vi "PulseIntervalHistogram_Relative.vi"(7 "Binary array reference":bool[](array[boolean]), 8 "Pulse count in":u64, 9 "No of SI bins":dbl=50.0, 11 "Binary array probe":bool[](array[boolean])) -> (0 "Pulse count out":u64, 1 "Pulse histogram":T1(graph), 2 "Pulse length histogram":T1(graph), 3 "Pulse period histogram":T1(graph))   [LabVIEW 2012]
uses:
  <vilib>/Analysis/NI_AALPro.lvlib
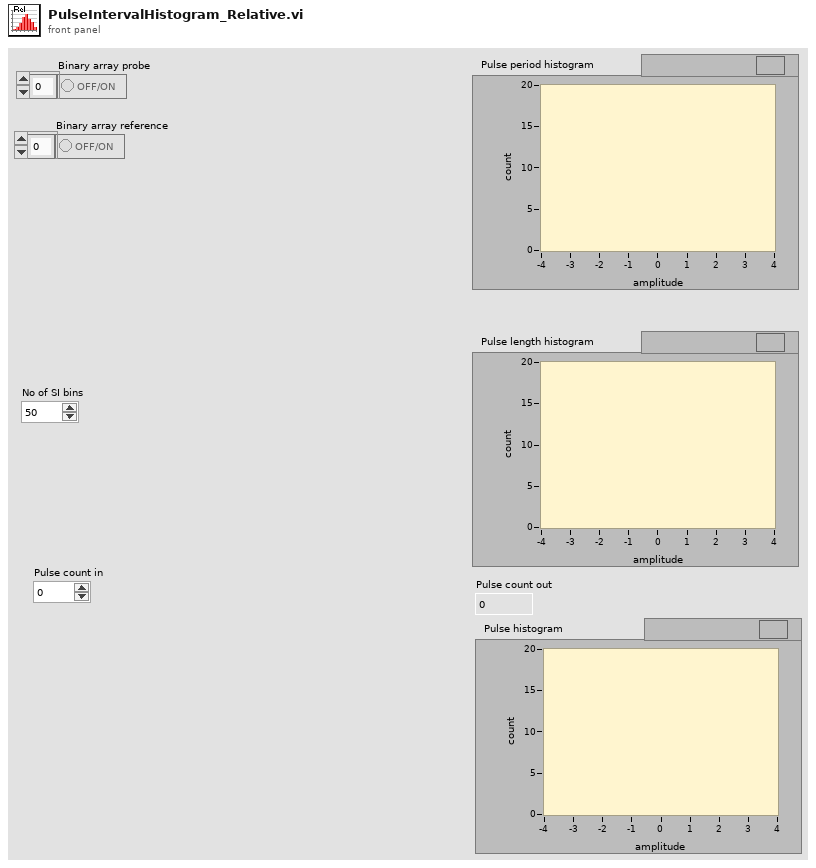
[diagram p1: front panel]
types:
  T1 = cluster{"X Values":dbl[], "Histogram: h(x)":i32[]}
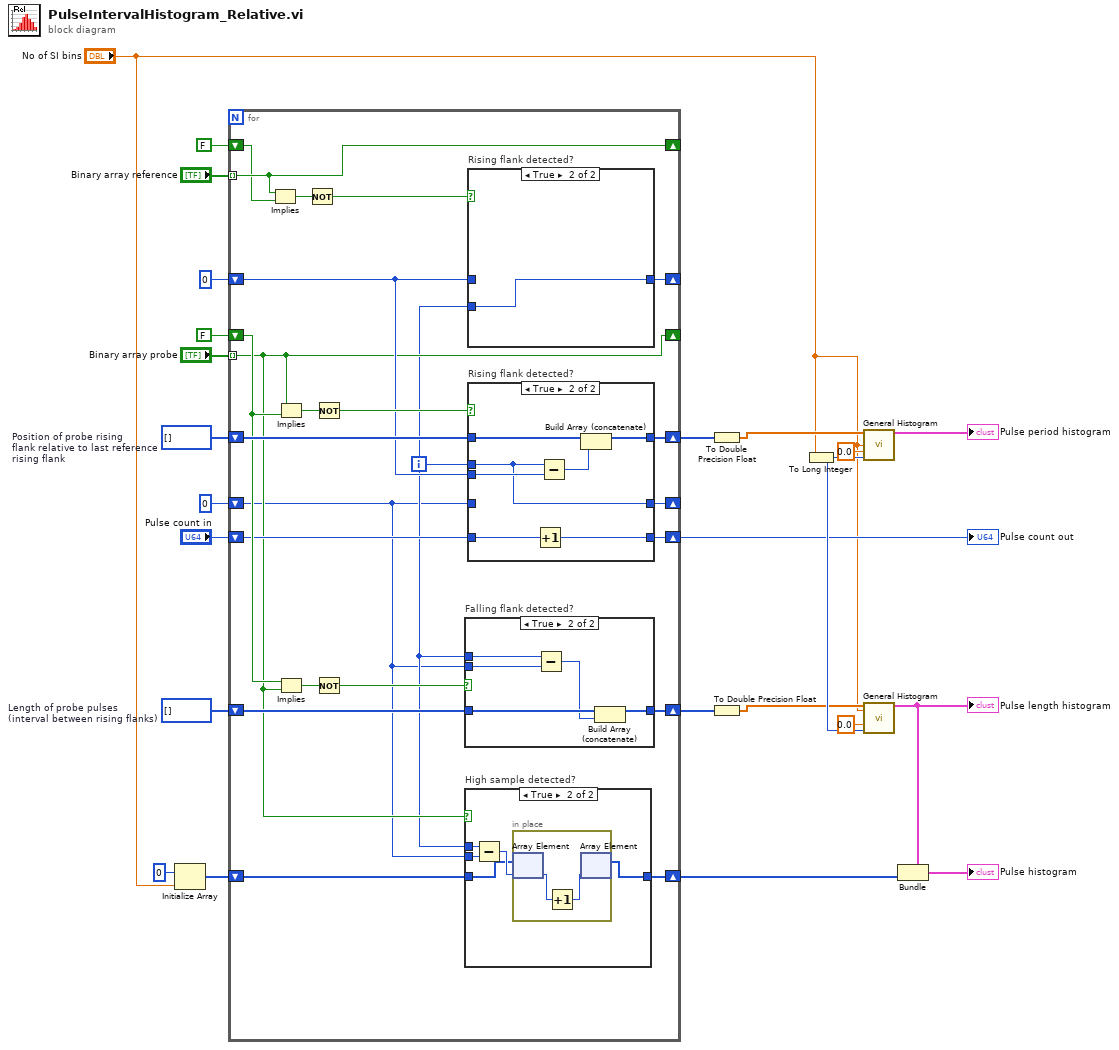
[diagram p0: block diagram]
diagram:
  w19 = i32[] []  # Length of probe pulses (interval between rising flanks)
  w22 = i32[] []  # Position of probe rising flank relative to last reference rising flank
  n1 = Initialize Array(0 ("element"), "No of SI bins") -> (w4:i32[])
  n2 = for {
    tunnel: "Binary array probe" -> [w29] mode=indexing
    shift-right: [w29] -> _
    shift-left: FALSE -> [w43]
    shift-right: [w45] -> w21
    shift-left: w22 -> [w44]
    shift-right: [w39] -> w18
    shift-left: w19 -> [w40]
    shift-right: [w37] -> w15
    shift-left: "Pulse count in" -> [w38]
    tunnel: "Binary array reference" -> [w36] mode=indexing
    shift-right: [w36] -> _
    shift-left: FALSE -> [w35]
    shift-right: [w32] -> _
    shift-left: 0 -> [w31]
    shift-right: [w30] -> _
    shift-left: 0 -> [w27]
    shift-right: [w25] -> w2
    shift-left: w4 -> [w26]
    i -> [w28]
    n3 = Implies(1:w35, 2:w36) -> (0:w34:bool)
    n4 = Implies(1:w43, 2:w29) -> (0:w47:bool)
    n5 = Implies(1:w29, 2:w43) -> (0:w42:bool)
    n6 = Not(x=w34) -> (.not. x?=w33:bool)
    n7 = Not(x=w47) -> (.not. x?=w46:bool)
    n8 = Not(x=w42) -> (.not. x?=w41:bool)
    n9 = case "Falling flank detected?" shown="True" w41 {
      tunnel: w40 -> [w58 w62]
      tunnel: w28 -> [_ w63]
      tunnel: [w58 w60] -> w39
      tunnel: w27 -> [_ w59]
      frame False {
      }
      frame True {
        n10 = Subtract(x=w63, y=w59) -> (x-y=w61:i32)
        n11 = Build Array (concatenate)(w62, w61) -> (w60:i32[])
      }
    }
    n12 = case "High sample detected?" shown="True" w29 {
      tunnel: w28 -> [_ w53]
      tunnel: w27 -> [_ w52]
      tunnel: w26 -> [w48 w50]
      tunnel: [w48 w49] -> w25
      frame False {
      }
      frame True {
        n13 = Subtract(x=w53, y=w52) -> (x-y=w51:i32)
        n14 = in-place {
          n15 = in-place-array #1(w50, w51) -> (w55:i32)
          n16 = Increment(x=w55) -> (x+1=w54:i32)
          n17 = in-place-array #1(w54) -> (w49:i32[])  [unwired: 1 out]
        }
      }
    }
    n18 = case "Rising flank detected?" shown="True" w33 {
      tunnel: w28 -> [_ w57]
      tunnel: [w56 w57] -> w32
      tunnel: w31 -> [w56 _]
      frame False {
      }
      frame True {
      }
    }
    n19 = case "Rising flank detected?" shown="True" w46 {
      tunnel: w28 -> [_ w67]
      tunnel: [w66 w72] -> w45
      tunnel: w44 -> [w66 w71]
      tunnel: w38 -> [w65 w70]
      tunnel: [w65 w69] -> w37
      tunnel: w31 -> [_ w68]
      tunnel: w27 -> [w64 _]
      tunnel: [w64 w67] -> w30
      frame False {
      }
      frame True {
        n20 = Increment(x=w70) -> (x+1=w69:u64)
        n21 = Subtract(x=w67, y=w68) -> (x-y=w73:i32)
        n22 = Build Array (concatenate)(w71, w73) -> (w72:i32[])
      }
    }
  }
  "Pulse count out" <- w15
  n23 = To Double Precision Float(number=w21) -> (double precision float=w10:dbl[])
  n24 = To Double Precision Float(number=w18) -> (double precision float=w9:dbl[])
  n25 = To Long Integer(number="No of SI bins") -> (32bit integer=w17:i32)
  n26 = call <vilib>:"General Histogram.vi"("X"=w10, "max"="No of SI bins", "min"=0.0, "# bins"=w17) -> ("Histogram Graph"=→"Pulse period histogram":T1)  [unwired: 7 in, 4 out]
  n27 = call <vilib>:"General Histogram.vi"("X"=w9, "max"="No of SI bins", "min"=0.0, "# bins"=w17) -> ("Histogram Graph"=w3:T1)  [unwired: 7 in, 4 out]
  "Pulse length histogram" <- w3
  n28 = Bundle(cluster=w3, "Histogram: h(x)"=w2) -> (→"Pulse histogram":T1)  [unwired: 1 in]
